vi "Zero oFF (SubVI).vi"(11 "Data":dbl[](array[numeric])) -> (3 "Array":dbl[](array[numeric]))   [LabVIEW 2014]
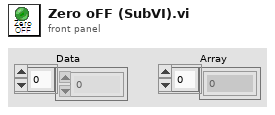
[diagram p1: front panel]
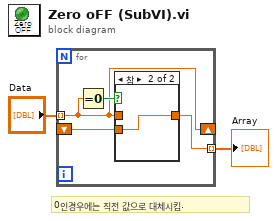
[diagram p0: block diagram]
diagram:
  # "0인경우에는 직전 값으로 대체시킴."
  n1 = for {
    tunnel: "Data" -> [w5] mode=indexing
    shift-right: [w5] -> _
    shift-left: _ -> [w3]
    tunnel: [w4] -> w2 mode=indexing
    n2 = Equal To 0?(x=w5) -> (x = 0?=w6:bool)
    n3 = case shown="참" w6 {
      tunnel: w5 -> [w7 _]
      tunnel: w3 -> [_ w8]
      tunnel: [w7 w8] -> w4
      frame False {
      }
      frame True {
      }
    }
  }
  "Array" <- w2
